vi "Init_Test.vi"(8 "error in (no error)":errorcluster caption="entrée d'erreur (pas d'erreur)", 11 "Get_Voltage en entrée":refnum<class "Wait_Frame_ERP1.lvclass">) -> (0 "error out":errorcluster caption="sortie d'erreur", 3 "Get_Voltage en sortie":refnum<class "Wait_Frame_ERP1.lvclass">)   [LabVIEW 2020, in "Library Test.lvlib" / "Wait_Frame_ERP1.lvclass"]
uses:
  Wait_Frame_ERP1.lvclass
  C:/Users/ngarcin/OneDrive - Altyor/Standard TB/Class/Test/Test (Default)/Test (Default).lvclass
  Commun VI/TypeDef/Commande Test/Commande Value Type.ctl
  Commun VI/TypeDef/Commande Test/Commande Type Test.ctl
  Test_Wtih_Instr/Test_With_Inst.lvclass
  Instrument/Instrument (Default)/Class Instrument (Default).lvclass
  Wait_Frame_ERP1.lvclass/Wait_Frame_ERP1.ctl
  Commun VI/Library Commun.lvlib
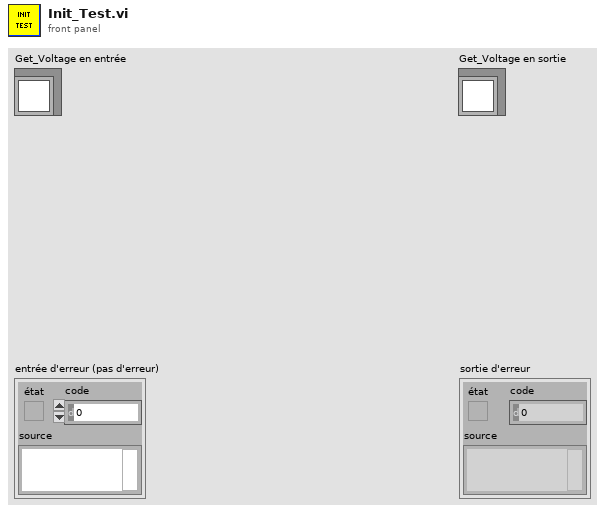
[diagram p1: front panel]
types:
  T1 = typedef "Library Commun.lvlib/Commande Type Test.ctl" = enum16{"Function", "Test", "Calculation"}
  T2 = typedef "Library Commun.lvlib/Commande Value Type.ctl" = enum16{"None", "String", "Number", "Timestamp", "Boolean", "Array"}
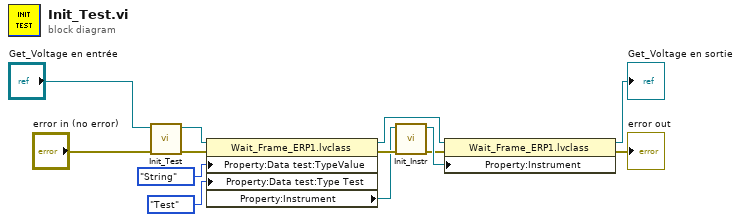
[diagram p0: block diagram]
diagram:
  n1 = call-parent "Init_Test.vi"("error in (no error)"="error in (no error)", "Test_With_Inst en entrée"="Get_Voltage en entrée") -> ("error out"=w10:errorcluster, "Test_With_Inst en sortie"=w11:refnum<class "Wait_Frame_ERP1.lvclass">)  [unwired: 8 in]
  n2 = property class="Wait_Frame_ERP1.lvclass"(reference=w11, error in=w10, "Property:Data test:TypeValue"=Commande_Value_Type."String" ("TypeValue"), "Property:Data test:Type Test"=Commande_Type_Test."Test" ("Type Test")) -> (reference out=w4:refnum<class "Wait_Frame_ERP1.lvclass">, error out=w7:errorcluster, "Property:Instrument"=w6:refnum<class "Class Instrument (Default).lvclass">)
  n3 = call-dynamic "Init_Instr.vi"("error in (no error)"=w7, "Class Instrument (Default) en entrée"=w6) -> ("error out"=w1:errorcluster, "Class Instrument (Default) en sortie"=w5:refnum<class "Class Instrument (Default).lvclass">)  [unwired: 8 in]
  n4 = property class="Wait_Frame_ERP1.lvclass"(reference=w4, error in=w1, "Property:Instrument"=w5) -> (reference out=→"Get_Voltage en sortie":refnum<class "Wait_Frame_ERP1.lvclass">, error out=→"error out":errorcluster)
